vi "ReadAdsState.vi"(8 "error in (no error)":errorcluster, 11 "AdsNET in":refnum<class "AdsNET.lvclass">) -> (0 "error out":errorcluster, 2 "AdsState":i16(ring) items=["Invalid", "Idle", "Reset", "Init", "Start", "Run", "Stop", "SaveConfig", "LoadConfig", "PowerFailure", "PowerGood", "Error", "Shutdown", "Suspend", "Resume", "Config", "Reconfig", "Maxstates"], 3 "AdsNET out":refnum<class "AdsNET.lvclass">)   [LabVIEW 2016, in "TCatAdsNet.lvlib" / "AdsNET.lvclass"]
doc: "Current state of the ADS device."
uses:
  AdsNET.lvclass
  AdsNET.lvclass/AdsNET.ctl
  C:/Users/Maurizio/Projects/twincat-lv-ads-library/TCatAdsNet Library/TwinCAT.Ads.dll
  TwinCAT.Ads.dll
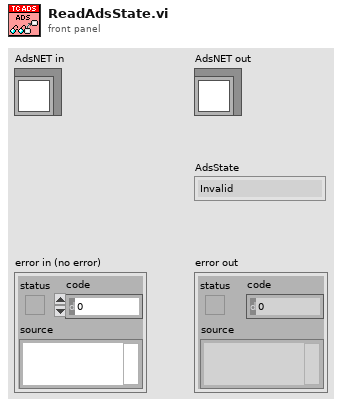
[diagram p1: front panel]
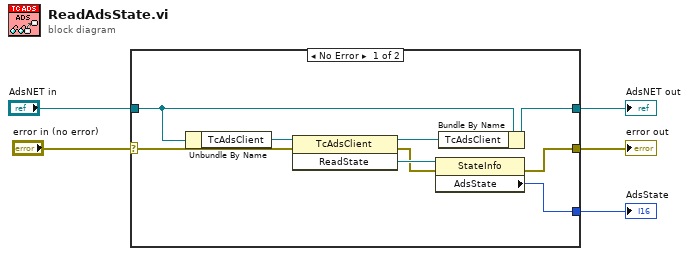
[diagram p0: block diagram]
diagram:
  n1 = case shown="No Error" "error in (no error)" {
    selector: "error in (no error)" -> [w12 w16]
    tunnel: [w7 w16] -> w4
    tunnel: [w11 w15] -> w2
    tunnel: "AdsNET in" -> [w14 w15]
    tunnel: [w6 _] -> w1
    frame No Error {
      n2 = Unbundle By Name(w14) -> ("TcAdsClient"=w13:refnum<k24>)
      n3 = invoke class="TcAdsClient" method="ReadState"(reference=w13, error in=w12) -> (reference out=w10:refnum<k24>, error out=w8:errorcluster, "ReadState"=w9:refnum<k24>)  [unwired: 1 in]
      n4 = property class="StateInfo"(reference=w9, error in=w8) -> (error out=w7:errorcluster, "AdsState"=w6:i16)  [unwired: 1 out]
      n5 = Bundle By Name(cluster=w14, "TcAdsClient"=w10) -> (w11:refnum<class "AdsNET.lvclass">)
    }
    frame Error {
    }
  }
  "error out" <- w4
  "AdsNET out" <- w2
  "AdsState" <- w1
